vi "Trigger_measurement.vi"(11 "VISA resource name":refnum<visa-resource-name>="COM4") -> (3 "Response":string)   [LabVIEW 2024]
doc: "This example performs writes and reads on a serial port, as directed by the user. You can press the Write and Read buttons, and change the Read Count, while the example is running.\n\nThe parameters set for the serial port must match the parameters of the connected instrument or device. In this example, the Read Count parameter specifies the number of bytes that the serial port reads. If there were more bytes at the port than the specified number, those bytes would not be read. If there were less bytes at the port than the specified number, you would receive a timeout error.\n\nThis example expands upon the flow control options for XON and XOFF, allowing the user to choose those control characters. Also, the user can enable or disable a termination character. Some devices require a termination character in order to identify the end of command strings. Some devices send a termination character to signify the end of data to be read. This example shows how you can end the Read operation once a termination character is detected in the buffer and/or append a termination character at the end of the Write data."
uses:
  support/Serial - XON-XOFF Characters.ctl
  support/Serial - ASCII Characters.ctl
  support/Serial - Settings.ctl
  <vilib>/Instr/_visa.llb/VISA Configure Serial Port (Instr).vi
panel:
  in  "String":string="Read?"
  in  "Read Count":u32=1000
  out "return count":u32=10
  # "Multi-Commands can be given in one command if seperated by semicolons"
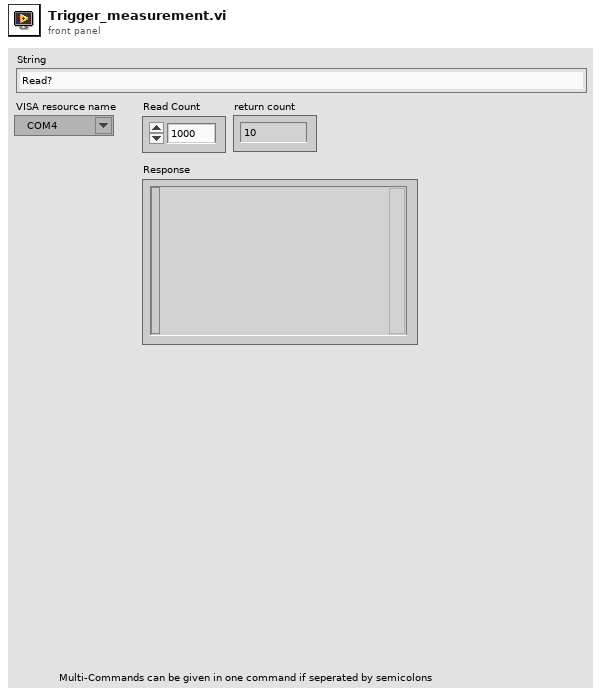
[diagram p1: front panel]
types:
  T1 = typedef "Serial - Settings.ctl" = cluster{"baud rate":u32, "data bits":u16, "parity":enum16{"None", "Odd", "Even", "Mark", "Space"}, "stop bits":u16, "flow control":u16}
  T2 = typedef "Serial - XON-XOFF Characters.ctl" = cluster{"XON":T3, "XOFF":T3}
  T3 = typedef "Serial - ASCII Characters.ctl" = enum16{"NUL", "SOH", "STX", "ETX", "EOT", "ENQ", "ACK", "BEL", "BS", "HT", "LF", "VT", "FF", "CR", "SO", "SI", "DLE", "DC1", "DC2", "DC3", "DC4", "NAK", "SYN", "ETB", "CAN", "EM", "SUB", "ESC", "FS", "GS", "RS", "US", "SP", "!", "\"", "#", "$", "%", "&", "'", "(", ")", "*", "+", ",", "- (-)", ".", "/", "0", "1", "2", "3", "4", "5", "6", "7", "8", "9", ":", ";", "<", "=", ">", "?", "@", "A", "B", "C", "D", "E", "F", "G", "H", "I", "J", "K", "L", "M", "N", "O", "P", "Q", "R", "S", "T", "U", "V", "W", "X", "Y", "Z", "[", "\\", "]", "^", "_", "`", "a", "b", "c", "d", "e", "f", "g", "h", "i", "j", "k", "l", "m", "n", "o", "p", "q", "r", "s", "t", "u", "v", "w", "x", "y", "z", "{", "|", "}", "~"}
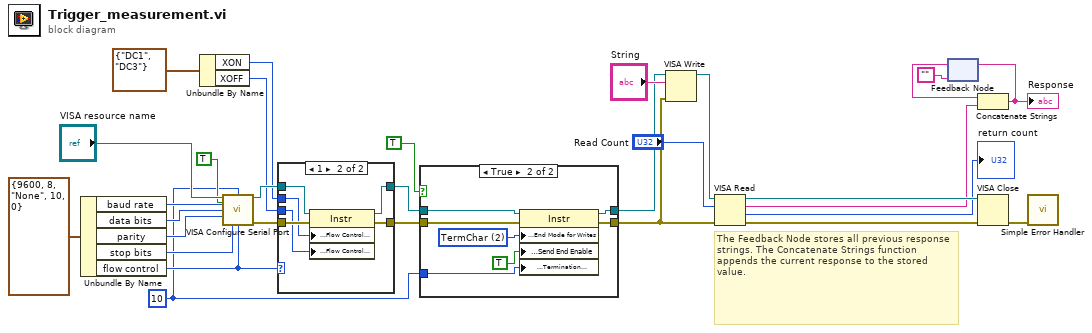
[diagram p0: block diagram]
diagram:
  w14 = u8 10 ("Termination Character")
  # "The Feedback Node stores all previous response strings. The Concatenate Strings function appends the current response to the stored value."
  n1 = Unbundle By Name(T1 {"baud rate"=9600, "data bits"=8, "parity"=enum."None", "stop bits"=10, "flow control"=0} ("Serial Settings")) -> ("baud rate"=w23:u32, "data bits"=w24:u16, "parity"=w25:enum16{"None", "Odd", "Even", "Mark", "Space"}, "stop bits"=w26:u16, "flow control"=w20:u16)
  n2 = Unbundle By Name(T2 {"XON"=enum."DC1", "XOFF"=enum."DC3"} ("XON/XOFF Characters")) -> ("XON"=w19:T3, "XOFF"=w18:T3)
  n3 = call-poly "VISA Configure Serial Port"("VISA resource name"="VISA resource name", "termination char\n(0xA = '\\n' = LF)"=w14, "Enable Termination\nChar (T)"=TRUE ("End Read on Termination Character?"), "baud rate (9600)"=w23, "data bits (8)"=w24, "parity (0:none)"=w25, "stop bits (10: 1 bit)"=w26, "flow control (0:none)"=w20) -> ("VISA resource name out"=w27:refnum<visa-resource-name>, "error out"=w28:errorcluster)  [unwired: 2 in, 4 out]
  n4 = case shown="1" w20 {
    tunnel: [w31 w38] -> w17
    tunnel: [w32 w37] -> w16
    tunnel: w28 -> [w31 w36]
    tunnel: w27 -> [w32 w35]
    tunnel: w19 -> [_ w34]
    tunnel: w18 -> [_ w33]
    frame Default {
    }
    frame 1 {
      n5 = property class="Instr"(reference=w35, error in=w36, "Serial Settings:Flow Control XON Character"=w34, "Serial Settings:Flow Control XOFF Character"=w33) -> (reference out=w37:refnum<visa-resource-name>, error out=w38:errorcluster)
    }
  }
  n6 = case shown="True" TRUE ("End Write on Termination Character?") {
    tunnel: w16 -> [w39 w47]
    tunnel: w17 -> [w40 w46]
    tunnel: [w39 w45] -> w3
    tunnel: [w40 w44] -> w2
    tunnel: w14 -> [_ w42]
    frame False {
    }
    frame True {
      w43 = u16 2 items=["None", "LastBit", "TermChar", "Break"] ("Serial Settings:Serial End Mode for Writes")
      n7 = property class="Instr"(reference=w47, error in=w46, "Serial Settings:End Mode for Writes"=w43, "Message Based Settings:Send End Enable"=TRUE, "Message Based Settings:Termination Character"=w42) -> (reference out=w45:refnum<visa-resource-name>, error out=w44:errorcluster)
    }
  }
  n8 = VISA Write(VISA resource name=w3, write buffer="String", error in (no error)=w2) -> (VISA resource name out=w1:refnum<visa-resource-name>)  [unwired: 2 out]
  n9 = VISA Read(VISA resource name=w1, byte count="Read Count", error in (no error)=w2) -> (VISA resource name out=w11:refnum<visa-resource-name>, read buffer=w8:string, return count=→"return count":u32, error out=w12:errorcluster)
  n10 = feedback #1("") -> (w7:string)
  n11 = Concatenate Strings(w7, w8) -> (w6:string)
  "Response" <- w6
  n12 = feedback-in #1(w6) -> ()
  n13 = VISA Close(VISA resource name=w11, error in (no error)=w12) -> (error out=w13:errorcluster)
  n14 = call <vilib>:"Simple Error Handler.vi"("error in (no error)"=w13) -> ()  [unwired: 1 in, 8 out]
